vi "LimitAngle.vi"(4 "atacando contra":bool, 6 "XdoAttacker":dbl, 7 "YdoAttacker":dbl, 8 "error in (no error)":errorcluster, 9 "AnguloGol":dbl, 10 "Game":refnum<class "Game.lvclass">, 11 "PositionToReceivePassSkill in":refnum<class "PositionToReceivePassSkill.lvclass">) -> (0 "error out":errorcluster, 2 "Angulo Limite":dbl, 3 "PositionToReceivePassSkill out":refnum<class "PositionToReceivePassSkill.lvclass">)   [LabVIEW 2018, in "PositionToReceivePassSkill.lvclass"]
uses:
  PositionToReceivePassSkill.lvclass
  Game_class/Game.lvclass
  Game_class/Game.lvclass/Game.ctl
  Game_class/Read FieldRef.vi
  Field_class/Field.lvclass
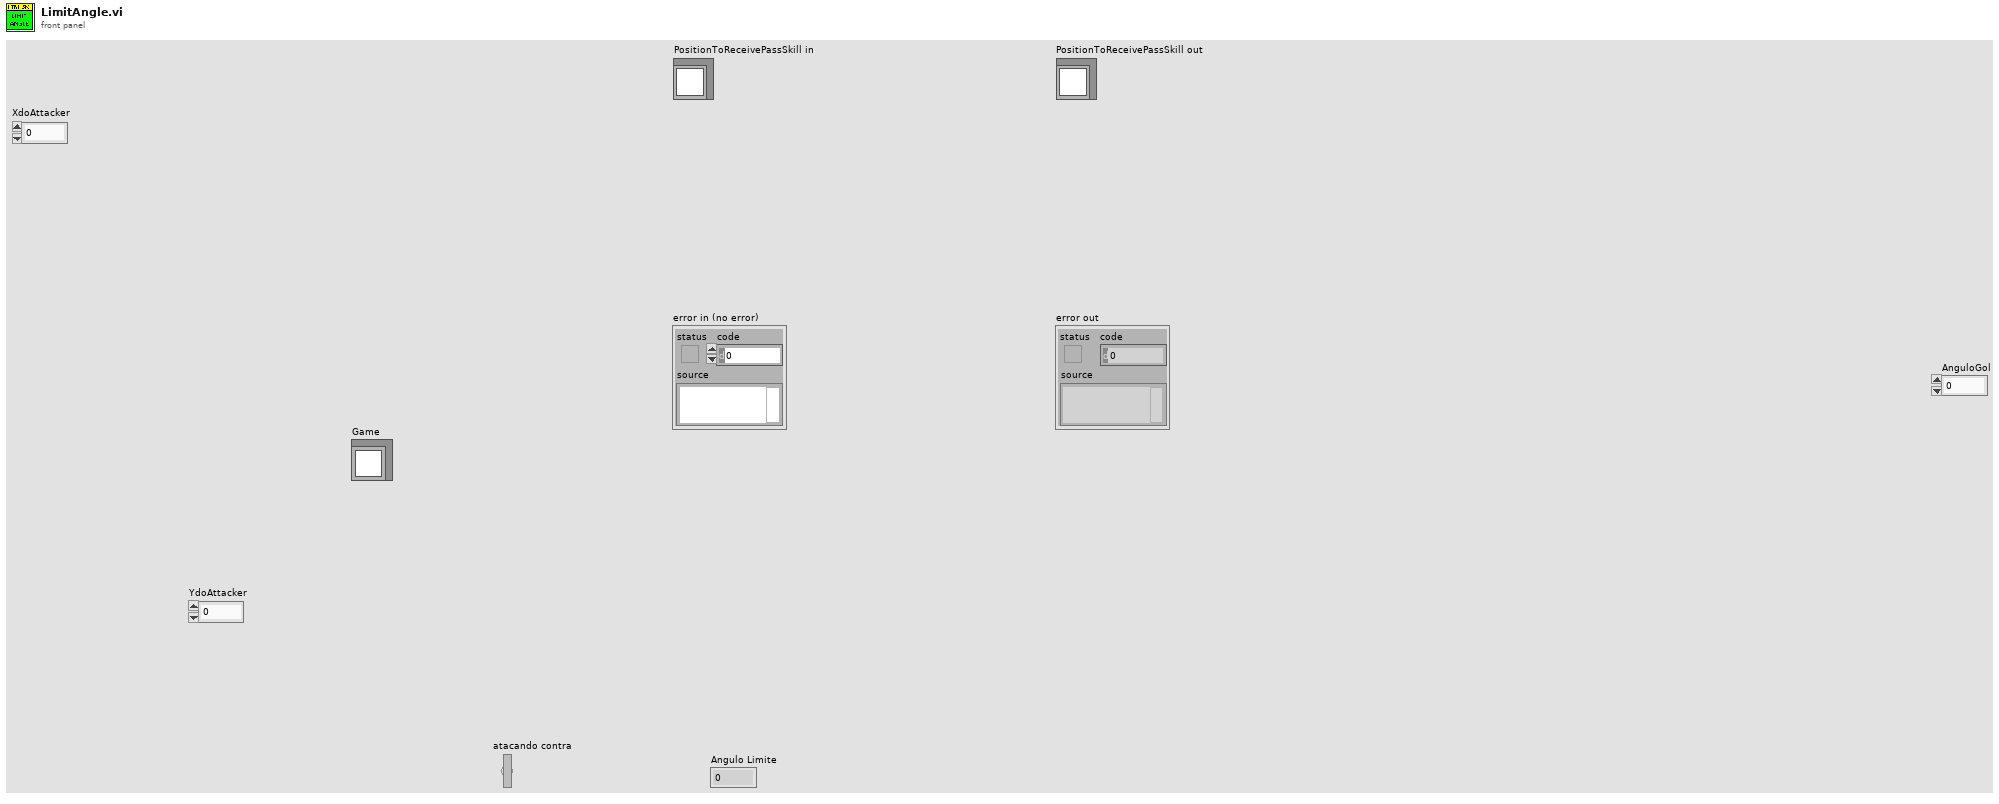
[diagram p1: front panel]
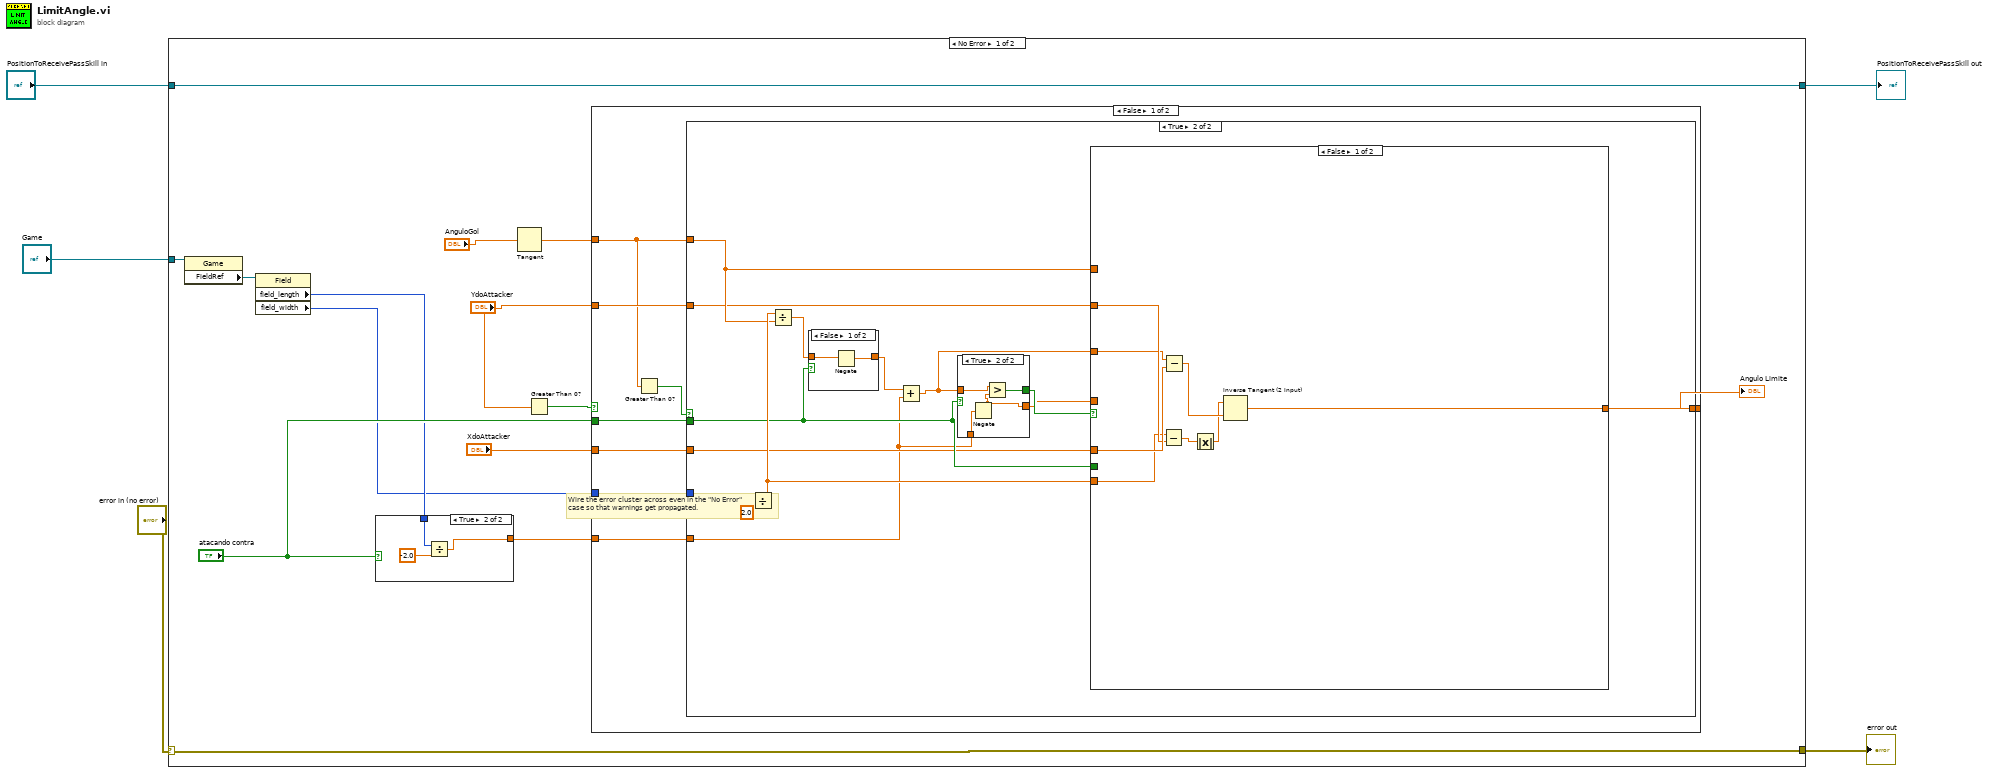
[diagram p0: block diagram]
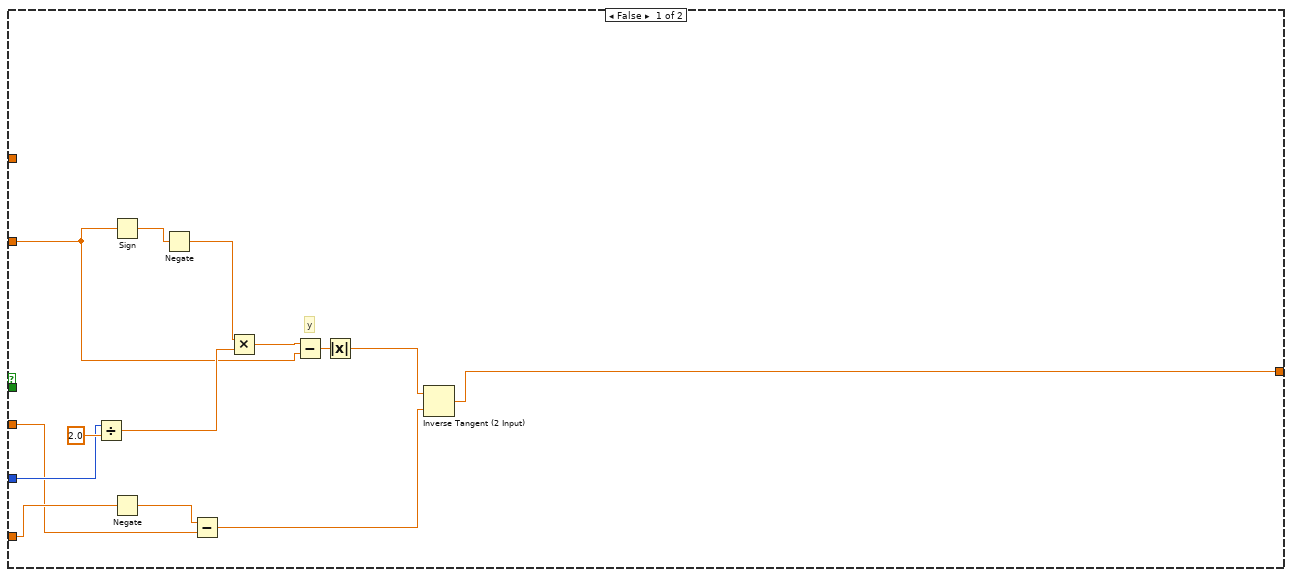
[diagram p2: hidden frame]
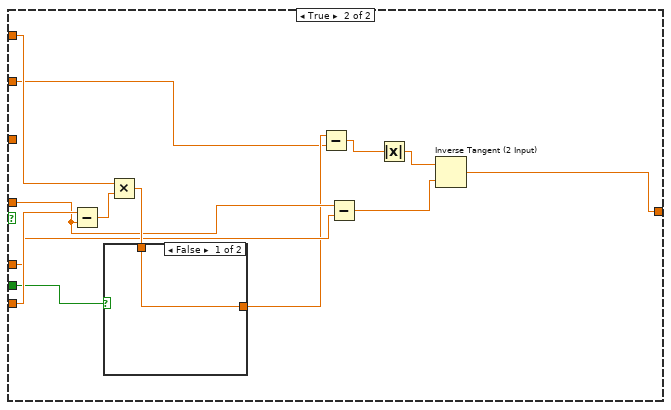
[diagram p3: hidden frame]
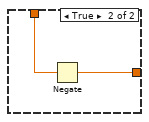
[diagram p4: hidden frame]
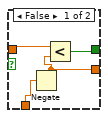
[diagram p5: hidden frame]
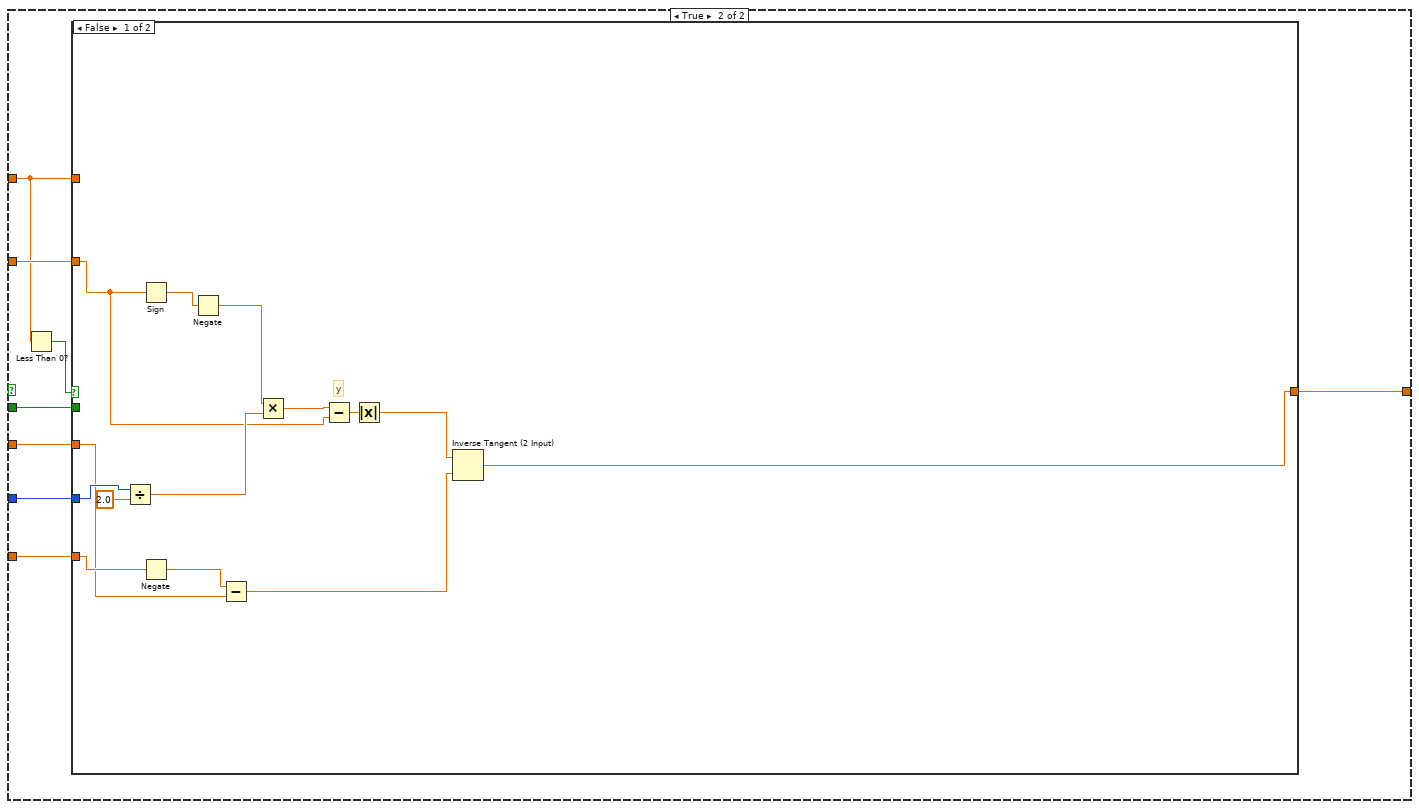
[diagram p7: hidden frame]
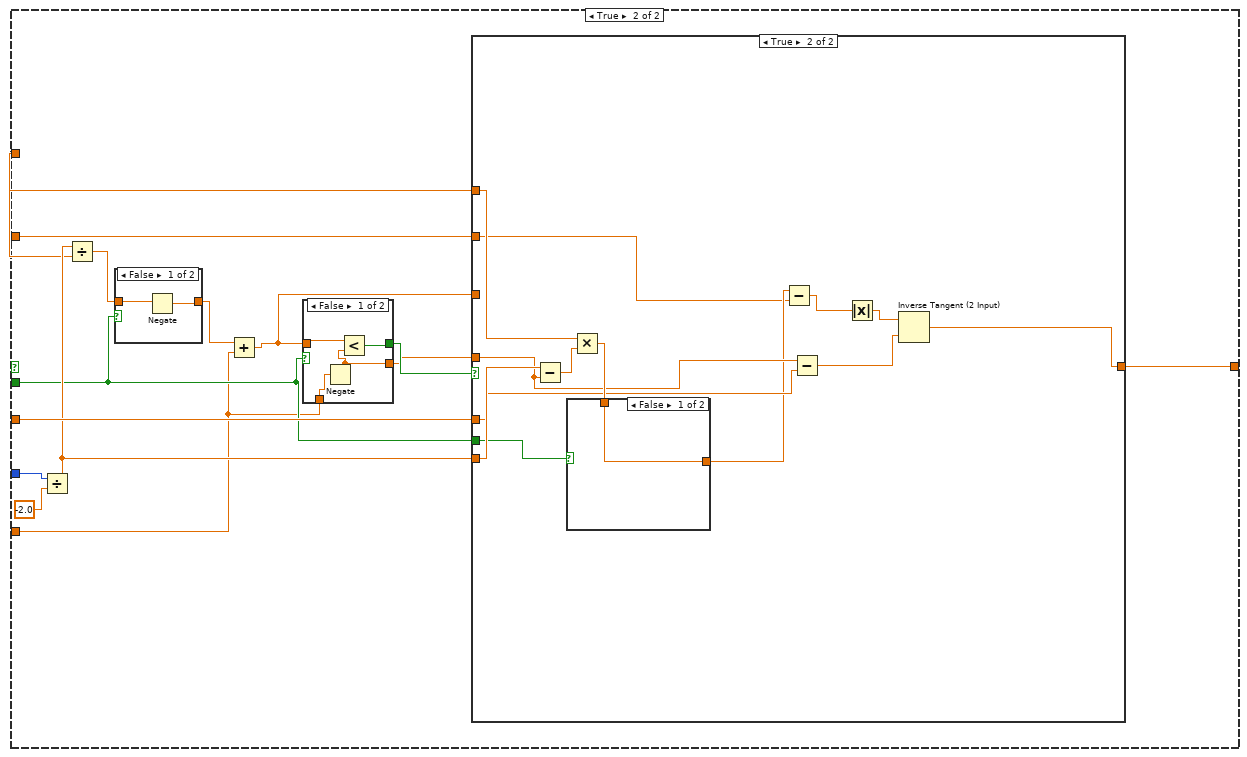
[diagram p8: hidden frame]
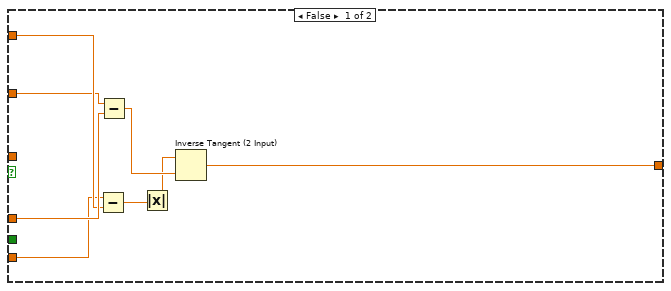
[diagram p9: hidden frame]
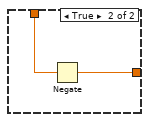
[diagram p10: hidden frame]
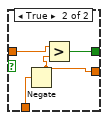
[diagram p11: hidden frame]
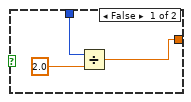
[diagram p13: hidden frame]
diagram:
  n1 = case shown="No Error" "error in (no error)" {
    selector: "error in (no error)" -> [w18 w169]
    tunnel: [w18 w169] -> w4
    tunnel: [w19 w168] -> w2
    tunnel: "PositionToReceivePassSkill in" -> [w19 w168]
    tunnel: "Game" -> [w9 _]
    frame No Error {
      # "Wire the error cluster across even in the \"No Error\"\ncase so that warnings get propagated."
      n2 = property class="Game"(reference=w9) -> ("FieldRef"=w8:refnum<class "Field.lvclass">)  [unwired: 1 in, 2 out]
      n3 = property class="Field"(reference=w8) -> ("field_length"=w7:i32, "field_width"=w6:i32)  [unwired: 1 in, 2 out]
      n4 = case shown="True" "atacando contra" {
        tunnel: w7 -> [w163 w167]
        tunnel: [w162 w165] -> w13
        frame False {
          n5 = Divide(x=w163, y=2.0) -> (x/y=w162:dbl)
        }
        frame True {
          n6 = Divide(x=w167, y=-2.0) -> (x/y=w165:dbl)
        }
      }
      n7 = Tangent(1:"AnguloGol") -> (0:w15:dbl)
      n8 = Greater Than 0?(x="YdoAttacker") -> (x > 0?=w17:bool)
      n9 = case shown="False" w17 {
        tunnel: w6 -> [w24 w98]
        tunnel: w15 -> [w22 w91]
        tunnel: "atacando contra" -> [w26 w94]
        tunnel: w13 -> [w23 w93]
        tunnel: "XdoAttacker" -> [w25 w97]
        tunnel: "YdoAttacker" -> [w27 w96]
        tunnel: [w20 w95] -> w10
        frame False {
          n10 = Greater Than 0?(x=w22) -> (x > 0?=w21:bool)
          n11 = case shown="True" w21 {
            tunnel: w22 -> [_ w48]
            tunnel: w27 -> [w32 w47]
            tunnel: w26 -> [_ w46]
            tunnel: w25 -> [w29 w45]
            tunnel: w24 -> [w31 w44]
            tunnel: w23 -> [w30 w43]
            tunnel: [w28 w42] -> w20
            frame False {
              # "y"
              n12 = Divide(x=w31, y=2.0) -> (x/y=w35:dbl)
              n13 = Sign(1:w32) -> (0:w33:dbl)
              n14 = Negate(x=w30) -> (-x=w38:dbl)
              n15 = Negate(x=w33) -> (-x=w36:dbl)
              n16 = Subtract(x=w38, y=w29) -> (x-y=w41:dbl)
              n17 = Multiply(x=w36, y=w35) -> (x*y=w37:dbl)
              n18 = Subtract(x=w37, y=w32) -> (x-y=w39:dbl)
              n19 = Absolute Value(x=w39) -> (abs(x)=w40:dbl)
              n20 = Inverse Tangent (2 Input)(1:w41, 2:w40) -> (0:w28:dbl)
            }
            frame True {
              n21 = Divide(x=w44, y=2.0) -> (x/y=w50:dbl)
              n22 = Divide(x=w50, y=w48) -> (x/y=w54:dbl)
              n23 = case shown="False" w46 {
                tunnel: w54 -> [w88 w90]
                tunnel: [w89 w90] -> w53
                frame False {
                  n24 = Negate(x=w88) -> (-x=w89:dbl)
                }
                frame True {
                }
              }
              n25 = Add(x=w53, y=w43) -> (x+y=w51:dbl)
              n26 = case shown="True" w46 {
                tunnel: w51 -> [w82 w87]
                tunnel: w43 -> [w83 w86]
                tunnel: [w81 w85] -> w52
                tunnel: [w80 w84] -> w49
                frame False {
                  n27 = Negate(x=w83) -> (-x=w80:dbl)
                  n28 = Less?(x=w82, y=w80) -> (x < y?=w81:bool)
                }
                frame True {
                  n29 = Negate(x=w86) -> (-x=w84:dbl)
                  n30 = Greater?(x=w87, y=w84) -> (0:w85:bool)
                }
              }
              n31 = case shown="False" w52 {
                tunnel: w45 -> [w63 w70]
                tunnel: w47 -> [w62 w68]
                tunnel: w51 -> [w61 _]
                tunnel: w50 -> [w60 w76]
                tunnel: [w58 w67] -> w42
                tunnel: w48 -> [_ w74]
                tunnel: w49 -> [_ w71]
                tunnel: w46 -> [_ w73]
                frame False {
                  n32 = Subtract(x=w60, y=w62) -> (x-y=w57:dbl)
                  n33 = Subtract(x=w61, y=w63) -> (x-y=w59:dbl)
                  n34 = Absolute Value(x=w57) -> (abs(x)=w56:dbl)
                  n35 = Inverse Tangent (2 Input)(1:w59, 2:w56) -> (0:w58:dbl)
                }
                frame True {
                  n36 = Subtract(x=w76, y=w71) -> (x-y=w75:dbl)
                  n37 = Multiply(x=w74, y=w75) -> (x*y=w72:dbl)
                  n38 = case shown="False" w73 {
                    tunnel: w72 -> [w77 w79]
                    tunnel: [w77 w78] -> w69
                    frame False {
                    }
                    frame True {
                      n39 = Negate(x=w79) -> (-x=w78:dbl)
                    }
                  }
                  n40 = Subtract(x=w69, y=w68) -> (x-y=w65:dbl)
                  n41 = Subtract(x=w71, y=w70) -> (x-y=w66:dbl)
                  n42 = Absolute Value(x=w65) -> (abs(x)=w64:dbl)
                  n43 = Inverse Tangent (2 Input)(1:w66, 2:w64) -> (0:w67:dbl)
                }
              }
            }
          }
        }
        frame True {
          n44 = Less Than 0?(x=w91) -> (x < 0?=w92:bool)
          n45 = case shown="False" w92 {
            tunnel: w98 -> [w110 w126]
            tunnel: w97 -> [w103 w121]
            tunnel: w96 -> [w105 w120]
            tunnel: [w99 w117] -> w95
            tunnel: w91 -> [_ w116]
            tunnel: w94 -> [_ w114]
            tunnel: w93 -> [w107 w113]
            frame False {
              # "y"
              n46 = Divide(x=w110, y=2.0) -> (x/y=w109:dbl)
              n47 = Sign(1:w105) -> (0:w112:dbl)
              n48 = Negate(x=w107) -> (-x=w104:dbl)
              n49 = Negate(x=w112) -> (-x=w108:dbl)
              n50 = Subtract(x=w104, y=w103) -> (x-y=w100:dbl)
              n51 = Multiply(x=w108, y=w109) -> (x*y=w106:dbl)
              n52 = Subtract(x=w106, y=w105) -> (x-y=w102:dbl)
              n53 = Absolute Value(x=w102) -> (abs(x)=w101:dbl)
              n54 = Inverse Tangent (2 Input)(1:w100, 2:w101) -> (0:w99:dbl)
            }
            frame True {
              n55 = Divide(x=w126, y=-2.0) -> (x/y=w118:dbl)
              n56 = Divide(x=w118, y=w116) -> (x/y=w124:dbl)
              n57 = case shown="False" w114 {
                tunnel: w124 -> [w159 w161]
                tunnel: [w160 w161] -> w123
                frame False {
                  n58 = Negate(x=w159) -> (-x=w160:dbl)
                }
                frame True {
                }
              }
              n59 = Add(x=w123, y=w113) -> (x+y=w119:dbl)
              n60 = case shown="False" w114 {
                tunnel: w119 -> [w153 w158]
                tunnel: w113 -> [w154 w157]
                tunnel: [w152 w156] -> w122
                tunnel: [w151 w155] -> w115
                frame False {
                  n61 = Negate(x=w154) -> (-x=w151:dbl)
                  n62 = Less?(x=w153, y=w151) -> (x < y?=w152:bool)
                }
                frame True {
                  n63 = Negate(x=w157) -> (-x=w155:dbl)
                  n64 = Greater?(x=w158, y=w155) -> (0:w156:bool)
                }
              }
              n65 = case shown="True" w122 {
                tunnel: w121 -> [w134 w141]
                tunnel: w120 -> [w133 w139]
                tunnel: w119 -> [w132 _]
                tunnel: w118 -> [w131 w147]
                tunnel: [w129 w138] -> w117
                tunnel: w116 -> [_ w145]
                tunnel: w115 -> [_ w142]
                tunnel: w114 -> [_ w144]
                frame False {
                  n66 = Subtract(x=w131, y=w133) -> (x-y=w128:dbl)
                  n67 = Subtract(x=w132, y=w134) -> (x-y=w130:dbl)
                  n68 = Absolute Value(x=w128) -> (abs(x)=w127:dbl)
                  n69 = Inverse Tangent (2 Input)(1:w130, 2:w127) -> (0:w129:dbl)
                }
                frame True {
                  n70 = Subtract(x=w147, y=w142) -> (x-y=w146:dbl)
                  n71 = Multiply(x=w145, y=w146) -> (x*y=w143:dbl)
                  n72 = case shown="False" w144 {
                    tunnel: w143 -> [w148 w150]
                    tunnel: [w148 w149] -> w140
                    frame False {
                    }
                    frame True {
                      n73 = Negate(x=w150) -> (-x=w149:dbl)
                    }
                  }
                  n74 = Subtract(x=w140, y=w139) -> (x-y=w135:dbl)
                  n75 = Subtract(x=w142, y=w141) -> (x-y=w137:dbl)
                  n76 = Absolute Value(x=w135) -> (abs(x)=w136:dbl)
                  n77 = Inverse Tangent (2 Input)(1:w137, 2:w136) -> (0:w138:dbl)
                }
              }
            }
          }
        }
      }
      "Angulo Limite" <- w10
    }
    frame Error {
    }
  }
  "error out" <- w4
  "PositionToReceivePassSkill out" <- w2
